vi "Register.vi"(8 "error in (no error)":errorcluster, 11 "Process Builder Model in":refnum<class "Process Builder Model.lvclass">) -> (0 "error out":errorcluster, 3 "Process Builder Model out":refnum<class "Process Builder Model.lvclass">)   [LabVIEW 2019, in "Process Builder Model.lvclass"]
uses:
  <vilib>/gpm_packages/@cs/Car-wash/Source/Process Builder Model/Process Builder Model.lvclass
  C:/Program Files/National Instruments/LabVIEW 2019/vi.lib/gpm_packages/@cs/mva-core/Source/IObserver/IObserver/IObserver.lvclass
  <vilib>/gpm_packages/@cs/Test-executive-builder/Source/Test Executive Builder Model/Test Executive Builder Model Messages/Load Test Executive Msg/Load Test Executive Msg.lvclass
  C:/Program Files/National Instruments/LabVIEW 2019/vi.lib/gpm_packages/@cs/transport/Source/Concrete/ActorMessageTransport/Notification Msg/Notification Msg.lvclass
  <vilib>/gpm_packages/@cs/mva-core/Source/SubscriptionPolicy/BasicSubscription/BasicSubscription.lvclass
  C:/Program Files/National Instruments/LabVIEW 2019/vi.lib/gpm_packages/@cs/mva-core/Source/IMediator/ISubscriptionPolicy/ISubscriptionPolicy.lvclass
  <vilib>/gpm_packages/@cs/Test-executive-builder/Source/Test Executive Builder Model/Test Executive Builder Model Messages/Insert While Loop Msg/Insert While Loop Msg.lvclass
  <vilib>/gpm_packages/@cs/Test-executive-builder/Source/Application Dependencies/Insert While Loop.ctl
  <vilib>/gpm_packages/@cs/Test-executive-builder/Source/Test Executive Builder Model/Test Executive Builder Model Messages/Insert For Loop Msg/Insert For Loop Msg.lvclass
  <vilib>/gpm_packages/@cs/Test-executive-builder/Source/Application Dependencies/Insert For Loop.ctl
  <vilib>/gpm_packages/@cs/Test-executive-builder/Source/Test Executive Builder Model/Test Executive Builder Model Messages/Insert Stop Loop Msg/Insert Stop Loop Msg.lvclass
  <vilib>/gpm_packages/@cs/Test-executive-builder/Source/Application Dependencies/Insert Stop Loop.ctl
  <vilib>/gpm_packages/@cs/Test-executive-builder/Source/Test Executive Builder Model/Test Executive Builder Model Messages/Insert Test Step Msg/Insert Test Step Msg.lvclass
  <vilib>/gpm_packages/@cs/Test-executive-builder/Source/Application Dependencies/Insert Test Step.ctl
  <vilib>/gpm_packages/@cs/Test-executive-builder/Source/Test Executive Builder Model/Test Executive Builder Model Messages/Insert Subroutine Msg/Insert Subroutine Msg.lvclass
  <vilib>/gpm_packages/@cs/Test-executive-builder/Source/Application Dependencies/Insert Subroutine.ctl
  <vilib>/gpm_packages/@cs/Test-executive-builder/Source/Test Executive Builder Model/Test Executive Builder Model Messages/Insert Subsequence Msg/Insert Subsequence Msg.lvclass
  <vilib>/gpm_packages/@cs/Test-executive-builder/Source/Application Dependencies/Insert Subsequence.ctl
  <vilib>/gpm_packages/@cs/Test-executive-builder/Source/Test Executive Builder Model/Test Executive Builder Model Messages/Insert Conditional Msg/Insert Conditional Msg.lvclass
  <vilib>/gpm_packages/@cs/Test-executive-builder/Source/Application Dependencies/Insert Conditional.ctl
  <vilib>/gpm_packages/@cs/Test-executive-builder/Source/Test Executive Builder Model/Test Executive Builder Model Messages/Remove Element Msg/Remove Element Msg.lvclass
  <vilib>/gpm_packages/@cs/Test-executive-builder/Source/Test Executive Builder Model/Test Executive Builder Model Messages/Move or Copy Element Msg/Move or Copy Element Msg.lvclass
  <vilib>/gpm_packages/@cs/Test-executive-builder/Source/Application Dependencies/Move or Copy Element.ctl
  <vilib>/gpm_packages/@cs/Test-executive-builder/Source/Test Executive Builder Model/Test Executive Builder Model Messages/Save Test Executive Msg/Save Test Executive Msg.lvclass
  <vilib>/gpm_packages/@cs/Test-executive-builder/Source/Test Executive Builder Model/Test Executive Builder Model Messages/Clear Test Executive Msg/Clear Test Executive Msg.lvclass
  <vilib>/gpm_packages/@cs/Test-executive-builder/Source/Test Executive Builder Model/Test Executive Builder Model Messages/Create Test Executive Msg/Create Test Executive Msg.lvclass
  <vilib>/gpm_packages/@cs/Test-executive-builder/Source/Application Dependencies/Create Test Executive.ctl
  <vilib>/gpm_packages/@cs/Test-executive-builder/Source/Test Executive Builder Model/Test Executive Builder Model Messages/Handle Double Click on Element Msg/Handle Double Click on Element Msg.lvclass
  <vilib>/gpm_packages/@cs/Test-executive-builder/Source/Test Executive Builder Model/Test Executive Builder Model Messages/Drop Element Msg/Drop Element Msg.lvclass
  <vilib>/gpm_packages/@cs/Test-executive-builder/Source/Application Dependencies/Drop Element.ctl
  <vilib>/gpm_packages/@cs/mva-core/Source/SubscriptionPolicy/BasicSubscription/BasicSubscription.lvclass/BasicSubscription.ctl
  <vilib>/ActorFramework/Actor/Actor.lvclass/Actor.ctl
  <vilib>/ActorFramework/Message Enqueuer/Message Enqueuer.lvclass/Message Enqueuer.ctl
  <vilib>/gpm_packages/@cs/transport/Source/Concrete/ActorMessageTransport/ActorMessageTransport.lvclass/ActorMessageTransport.ctl
  <vilib>/gpm_packages/@cs/mva-core/Source/IMediator/SubscriptionRequest/SubscriptionRequest.lvclass/SubscriptionRequest.ctl
  <vilib>/gpm_packages/@cs/mva-core/Source/IObserver/IObserver Messages/Subscribe Msg/Subscribe Msg.lvclass/Subscribe Msg.ctl
  <vilib>/gpm_packages/@cs/Car-wash/Source/Process Builder Model/Process Builder Model.lvclass/Process Builder Model.ctl
  <vilib>/gpm_packages/@cs/mva-core/Source/IMediator/SubscriptionRequest/Pack Subscription Request.vi
  <vilib>/gpm_packages/@cs/mva-core/Source/IObserver/IObserver Messages/Subscribe Msg/Send Subscribe.vi
  <vilib>/ActorFramework/Actor/Read Self Enqueuer.vi
  <vilib>/gpm_packages/@cs/transport/Source/Concrete/ActorMessageTransport/Construct Actor Message Transport.vi
  <vilib>/ActorFramework/Message Enqueuer/Enqueue.vi
  <vilib>/ActorFramework/Message Enqueuer/Init from Existing Queue.vi
  <vilib>/ActorFramework/Message Enqueuer/Equals Not A Refnum.vi
  <vilib>/gpm_packages/@cs/mva-core/Source/IObserver/IObserver/IObserver.lvclass
  C:/Program Files/National Instruments/LabVIEW 2019/vi.lib/ActorFramework/Actor/Actor.lvclass
  <vilib>/gpm_packages/@cs/transport/Source/Concrete/ActorMessageTransport/ActorMessageTransport.lvclass
  C:/Program Files/National Instruments/LabVIEW 2019/vi.lib/gpm_packages/@cs/transport/Source/ITransport/ITransport.lvclass
  <vilib>/gpm_packages/@cs/mva-core/Source/IObserver/IObserver Messages/Subscribe Msg/Subscribe Msg.lvclass
  C:/Program Files/National Instruments/LabVIEW 2019/vi.lib/ActorFramework/Message/Message.lvclass
  <vilib>/Utility/error.llb/Error Cluster From Error Code.vi
  <vilib>/gpm_packages/@cs/mva-core/Source/IMediator/ISubscriptionPolicy/Open Subscription Policy.vi
  <vilib>/ActorFramework/Message Priority Queue/Priority Enqueue.vi
  <vilib>/ActorFramework/Message Enqueuer/Message Enqueuer.lvclass
  <vilib>/gpm_packages/@cs/mva-core/Source/IMediator/SubscriptionRequest/SubscriptionRequest.lvclass
  <vilib>/gpm_packages/@cs/transport/Source/Concrete/ActorMessageTransport/Notification Msg/Notification Msg.lvclass
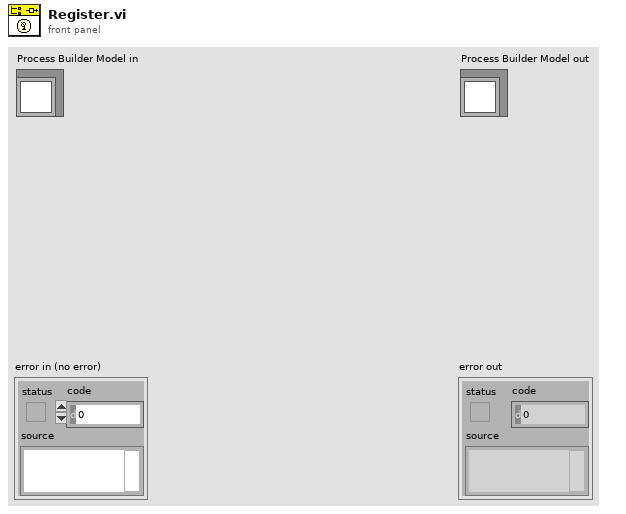
[diagram p1: front panel]
types:
  T1 = typedef "Drop Element.ctl" = cluster{"Parent ID":string, "Insertion Index":i32, "Tag":string, "Ctrl":bool}
  T2 = typedef "Create Test Executive.ctl" = cluster{"Folder Path":path, "File Name with Extension":string}
  T3 = typedef "Move or Copy Element.ctl" = cluster{"Parent ID":string, "Insertion Index":i32, "Tag":string, "Ctrl":bool}
  T4 = typedef "Insert Conditional.ctl" = cluster{"Parent ID":string, "Insertion Index":i32}
  T5 = typedef "Insert Subsequence.ctl" = cluster{"Parent ID":string, "Insertion Index":i32}
  T6 = typedef "Insert Subroutine.ctl" = cluster{"Parent ID":string, "Insertion Index":i32, "Path":path}
  T7 = typedef "Insert Test Step.ctl" = cluster{"Parent ID":string, "Insertion Index":i32, "Test Step":string}
  T8 = typedef "Insert Stop Loop.ctl" = cluster{"Parent ID":string, "Insertion Index":i32}
  T9 = typedef "Insert For Loop.ctl" = cluster{"Parent ID":string, "Insertion Index":i32, "Iterations":i32}
  T10 = typedef "Insert While Loop.ctl" = cluster{"Parent ID":string, "Insertion Index":i32}
  T11 = typedef "IMediator.lvlib/ISubscriptionPolicy.lvclass/ISubscriptionPolicy Reference.ctl" = refnum<data-value>
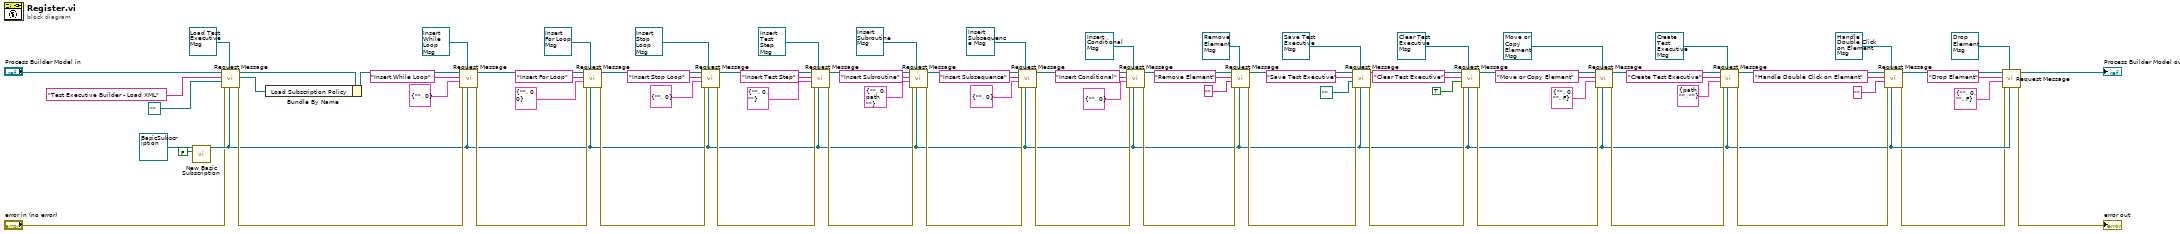
[diagram p0: block diagram]
diagram:
  n1 = call <vilib>:"New Basic Subscription.vi"("Ignore Past Updates? (F)"=FALSE, "BasicSubscription In"=refnum<class "BasicSubscription.lvclass"> refnum ("SubscriptionPolicy.lvlib:BasicSubscription.lvclass")) -> ("BasicSubscription Out"=w8:refnum<class "BasicSubscription.lvclass">)  [unwired: 9 in]
  n2 = call <vilib>:"Request Message.vi"("Configured SubscriptionPolicy"=w8, "Desired Notification Msg"=refnum<class "Load Test Executive Msg.lvclass"> refnum ("Load Test Executive Msg.lvclass"), "error in (no error)"="error in (no error)", "Data Type"=path "", "Datum Name"="Test Executive Builder - Load XML", "IObserver in"="Process Builder Model in") -> ("error out"=w75:errorcluster, "Subscription Policy"=w77:T11, "IObserver out"=w2:refnum<class "Process Builder Model.lvclass">)  [unwired: 3 in]
  n3 = Bundle By Name(cluster=w2, "Load Subscription Policy"=w77) -> (w1:refnum<class "Process Builder Model.lvclass">)
  n4 = call <vilib>:"Request Message.vi"("Configured SubscriptionPolicy"=w8, "Desired Notification Msg"=refnum<class "Insert While Loop Msg.lvclass"> refnum ("Insert While Loop Msg.lvclass"), "error in (no error)"=w75, "Data Type"=T10 {"Parent ID"="", "Insertion Index"=0} ("Insert While Loop"), "Datum Name"="Insert While Loop", "IObserver in"=w1) -> ("error out"=w68:errorcluster, "IObserver out"=w69:refnum<class "Process Builder Model.lvclass">)  [unwired: 3 in, 1 out]
  n5 = call <vilib>:"Request Message.vi"("Configured SubscriptionPolicy"=w8, "Desired Notification Msg"=refnum<class "Insert For Loop Msg.lvclass"> refnum ("Insert For Loop Msg.lvclass"), "error in (no error)"=w68, "Data Type"=T9 {"Parent ID"="", "Insertion Index"=0, "Iterations"=0} ("Insert For Loop"), "Datum Name"="Insert For Loop", "IObserver in"=w69) -> ("error out"=w63:errorcluster, "IObserver out"=w64:refnum<class "Process Builder Model.lvclass">)  [unwired: 3 in, 1 out]
  n6 = call <vilib>:"Request Message.vi"("Configured SubscriptionPolicy"=w8, "Desired Notification Msg"=refnum<class "Insert Stop Loop Msg.lvclass"> refnum ("Insert Stop Loop Msg.lvclass"), "error in (no error)"=w63, "Data Type"=T8 {"Parent ID"="", "Insertion Index"=0} ("Insert Stop Loop"), "Datum Name"="Insert Stop Loop", "IObserver in"=w64) -> ("error out"=w58:errorcluster, "IObserver out"=w59:refnum<class "Process Builder Model.lvclass">)  [unwired: 3 in, 1 out]
  n7 = call <vilib>:"Request Message.vi"("Configured SubscriptionPolicy"=w8, "Desired Notification Msg"=refnum<class "Insert Test Step Msg.lvclass"> refnum ("Insert Test Step Msg.lvclass"), "error in (no error)"=w58, "Data Type"=T7 {"Parent ID"="", "Insertion Index"=0, "Test Step"=""} ("Insert Test Step"), "Datum Name"="Insert Test Step", "IObserver in"=w59) -> ("error out"=w53:errorcluster, "IObserver out"=w54:refnum<class "Process Builder Model.lvclass">)  [unwired: 3 in, 1 out]
  n8 = call <vilib>:"Request Message.vi"("Configured SubscriptionPolicy"=w8, "Desired Notification Msg"=refnum<class "Insert Subroutine Msg.lvclass"> refnum ("Insert Subroutine Msg.lvclass"), "error in (no error)"=w53, "Data Type"=T6 {"Parent ID"="", "Insertion Index"=0, "Path"=path ""} ("Insert Subroutine"), "Datum Name"="Insert Subroutine", "IObserver in"=w54) -> ("error out"=w48:errorcluster, "IObserver out"=w49:refnum<class "Process Builder Model.lvclass">)  [unwired: 3 in, 1 out]
  n9 = call <vilib>:"Request Message.vi"("Configured SubscriptionPolicy"=w8, "Desired Notification Msg"=refnum<class "Insert Subsequence Msg.lvclass"> refnum ("Insert Subsequence Msg.lvclass"), "error in (no error)"=w48, "Data Type"=T5 {"Parent ID"="", "Insertion Index"=0} ("Insert Subsequence"), "Datum Name"="Insert Subsequence", "IObserver in"=w49) -> ("error out"=w43:errorcluster, "IObserver out"=w44:refnum<class "Process Builder Model.lvclass">)  [unwired: 3 in, 1 out]
  n10 = call <vilib>:"Request Message.vi"("Configured SubscriptionPolicy"=w8, "Desired Notification Msg"=refnum<class "Insert Conditional Msg.lvclass"> refnum ("Insert Conditional Msg.lvclass"), "error in (no error)"=w43, "Data Type"=T4 {"Parent ID"="", "Insertion Index"=0} ("Insert Conditional"), "Datum Name"="Insert Conditional", "IObserver in"=w44) -> ("error out"=w38:errorcluster, "IObserver out"=w39:refnum<class "Process Builder Model.lvclass">)  [unwired: 3 in, 1 out]
  n11 = call <vilib>:"Request Message.vi"("Configured SubscriptionPolicy"=w8, "Desired Notification Msg"=refnum<class "Remove Element Msg.lvclass"> refnum ("Remove Element Msg.lvclass"), "error in (no error)"=w38, "Data Type"="", "Datum Name"="Remove Element", "IObserver in"=w39) -> ("error out"=w25:errorcluster, "IObserver out"=w26:refnum<class "Process Builder Model.lvclass">)  [unwired: 3 in, 1 out]
  n12 = call <vilib>:"Request Message.vi"("Configured SubscriptionPolicy"=w8, "Desired Notification Msg"=refnum<class "Save Test Executive Msg.lvclass"> refnum ("Save Test Executive Msg.lvclass"), "error in (no error)"=w25, "Data Type"=path "", "Datum Name"="Save Test Executive", "IObserver in"=w26) -> ("error out"=w24:errorcluster, "IObserver out"=w34:refnum<class "Process Builder Model.lvclass">)  [unwired: 3 in, 1 out]
  n13 = call <vilib>:"Request Message.vi"("Configured SubscriptionPolicy"=w8, "Desired Notification Msg"=refnum<class "Clear Test Executive Msg.lvclass"> refnum ("Clear Test Executive Msg.lvclass"), "error in (no error)"=w24, "Data Type"=TRUE, "Datum Name"="Clear Test Executive", "IObserver in"=w34) -> ("error out"=w23:errorcluster, "IObserver out"=w33:refnum<class "Process Builder Model.lvclass">)  [unwired: 3 in, 1 out]
  n14 = call <vilib>:"Request Message.vi"("Configured SubscriptionPolicy"=w8, "Desired Notification Msg"=refnum<class "Move or Copy Element Msg.lvclass"> refnum ("Move or Copy Element Msg.lvclass"), "error in (no error)"=w23, "Data Type"=T3 {"Parent ID"="", "Insertion Index"=0, "Tag"="", "Ctrl"=FALSE} ("Move or Copy Element"), "Datum Name"="Move or Copy Element", "IObserver in"=w33) -> ("error out"=w20:errorcluster, "IObserver out"=w21:refnum<class "Process Builder Model.lvclass">)  [unwired: 3 in, 1 out]
  n15 = call <vilib>:"Request Message.vi"("Configured SubscriptionPolicy"=w8, "Desired Notification Msg"=refnum<class "Create Test Executive Msg.lvclass"> refnum ("Create Test Executive Msg.lvclass"), "error in (no error)"=w20, "Data Type"=T2 {"Folder Path"=path "", "File Name with Extension"=""} ("Create Test Executive"), "Datum Name"="Create Test Executive", "IObserver in"=w21) -> ("error out"=w13:errorcluster, "IObserver out"=w14:refnum<class "Process Builder Model.lvclass">)  [unwired: 3 in, 1 out]
  n16 = call <vilib>:"Request Message.vi"("Configured SubscriptionPolicy"=w8, "Desired Notification Msg"=refnum<class "Handle Double Click on Element Msg.lvclass"> refnum ("Handle Double Click on Element Msg.lvclass"), "error in (no error)"=w13, "Data Type"="", "Datum Name"="Handle Double Click on Element", "IObserver in"=w14) -> ("error out"=w7:errorcluster, "IObserver out"=w9:refnum<class "Process Builder Model.lvclass">)  [unwired: 3 in, 1 out]
  n17 = call <vilib>:"Request Message.vi"("Configured SubscriptionPolicy"=w8, "Desired Notification Msg"=refnum<class "Drop Element Msg.lvclass"> refnum ("Drop Element Msg.lvclass"), "error in (no error)"=w7, "Data Type"=T1 {"Parent ID"="", "Insertion Index"=0, "Tag"="", "Ctrl"=FALSE} ("Drop Element"), "Datum Name"="Drop Element", "IObserver in"=w9) -> ("error out"=→"error out":errorcluster, "IObserver out"=→"Process Builder Model out":refnum<class "Process Builder Model.lvclass">)  [unwired: 3 in, 1 out]
